vi "Event Driven Data Transfer.vi"() -> ()   [LabVIEW 2013]
uses:
  lightfield-automation-labview/LightField Automation.lvclass
panel:
  in  "ExperimentName":string
  out "Intensity Graph":dbl[][](graph)
  out "Time Per Loop":dbl
  out "Waveform Graph":dbl[](graph)
  out "# elements in queue":i32
  in  "stop":bool
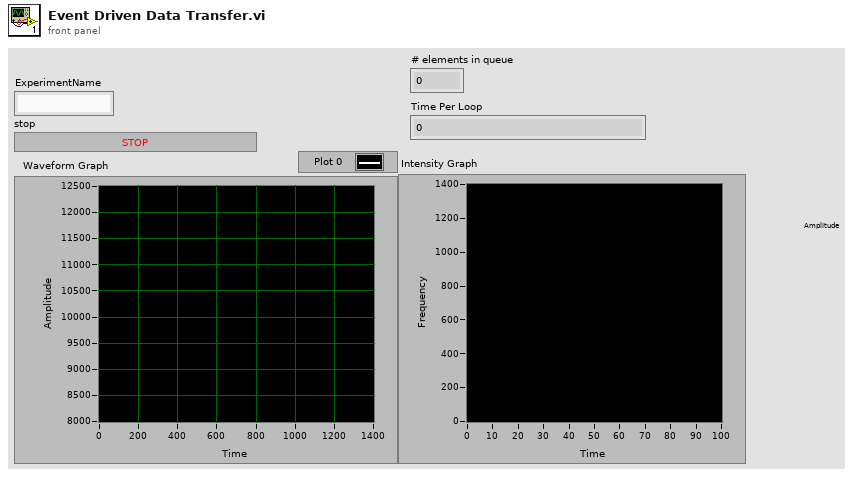
[diagram p1: front panel]
types:
  T1 = cluster{"Image":dbl[][][], "Frame Size":cluster{"F":i32, "Y":i32, "X":i32}}[]
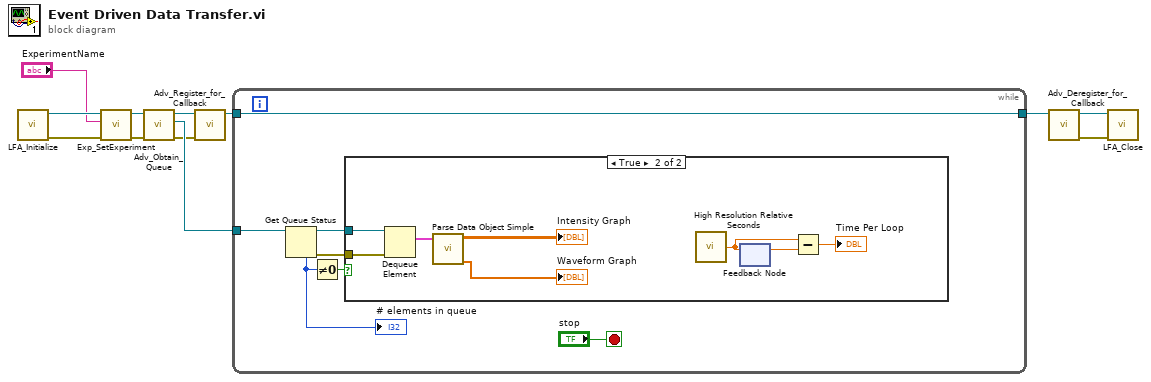
[diagram p0: block diagram]
diagram:
  n1 = call "LFA_Initialize.vi"() -> ("error out"=w5:errorcluster, "LightField Automation out"=w7:refnum<class "LightField Automation.lvclass">)  [unwired: 10 in]
  n2 = call "Exp_SetExperiment.vi"("error in (no error)"=w5, "ExperimentName"="ExperimentName", "LightField Automation in"=w7) -> ("error out"=w4:errorcluster, "LightField Automation out"=w6:refnum<class "LightField Automation.lvclass">)  [unwired: 7 in]
  n3 = call "Adv_Obtain_Queue.vi"("error in (no error)"=w4, "LightField Automation in"=w6) -> ("error out"=w10:errorcluster, "Queue Reference"=w11:refnum<queue>, "LightField Automation out"=w12:refnum<class "LightField Automation.lvclass">)  [unwired: 7 in]
  n4 = call "Adv_Register_for_Callback.vi"("error in (no error)"=w10, "LightField Automation in"=w12) -> ("LightField Automation out"=w9:refnum<class "LightField Automation.lvclass">)  [unwired: 8 in, 1 out]
  n5 = while {
    tunnel: w11 -> [w18]
    tunnel: w9 -> [w13]
    tunnel: [w13] -> w8
    stop <- "stop" stop-if-true
    n6 = Get Queue Status(queue=w18) -> (queue out=w17:refnum<queue>, error out=w16:errorcluster, # elements in queue=w14:i32)  [unwired: 2 in, 5 out]
    "# elements in queue" <- w14
    n7 = Not Equal To 0?(x=w14) -> (x != 0?=w15:bool)
    n8 = case shown="True" w15 {
      tunnel: w17 -> [_ w27]
      tunnel: w16 -> [_ w26]
      frame False {
      }
      frame True {
        n9 = Dequeue Element(queue=w27, error in (no error)=w26) -> (element=w22:T1)  [unwired: 1 in, 3 out]
        n10 = call "Parse Data Object Simple.vi"("Data"=w22) -> ("ROI 1, Frame 1, Row 1"=→"Waveform Graph":dbl[], "ROI 1, Frame 1"=→"Intensity Graph":dbl[][])  [unwired: 9 in]
        n11 = call <vilib>:"High Resolution Relative Seconds.vi"() -> ("relative seconds"=w24:dbl)
        n12 = feedback-in #1(w24) -> ()
        n13 = feedback #1() -> (w25:dbl)  [unwired: 1 in]
        n14 = Subtract(x=w24, y=w25) -> (x-y=→"Time Per Loop":dbl)
      }
    }
  }
  n15 = call "Adv_Deregister_for_Callback.vi"("LightField Automation in"=w8) -> ("error out"=w2:errorcluster, "LightField Automation out"=w1:refnum<class "LightField Automation.lvclass">)  [unwired: 9 in]
  n16 = call "LFA_Close.vi"("error in (no error)"=w2, "LightField Automation in"=w1) -> ()  [unwired: 8 in, 2 out]
